vi "ConvertToWriteByte.vi"(1 "Input":u16) -> (0 "Output":u16)   [LabVIEW 2016, in "FPGAMockMDILC.lvlib"]
uses:
  FPGAMockMDILC.lvlib
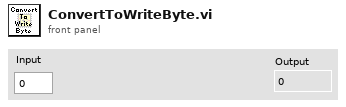
[diagram p1: front panel]
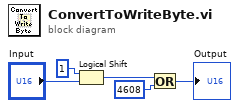
[diagram p0: block diagram]
diagram:
  n1 = Logical Shift(y=i16 1, x="Input") -> (x << y=w3:u16)
  n2 = Or(x=w3, y=u16 4608) -> (x .or. y?=→"Output":u16)
